vi "Prueba_report.vi"() -> ()   [LabVIEW 2025]
panel:
  out "Waveform Chart":dbl(graph)
  out "Waveform Graph":dbl[](graph)
  in  "stop":bool
  out "error out":errorcluster
  in  "error in (no error)":errorcluster
  in  "Canal 3":string
  in  "Canal 2":string
  in  "Canal 1":string
  in  "Grupo":string
  in  "Cantidad de datos":i32
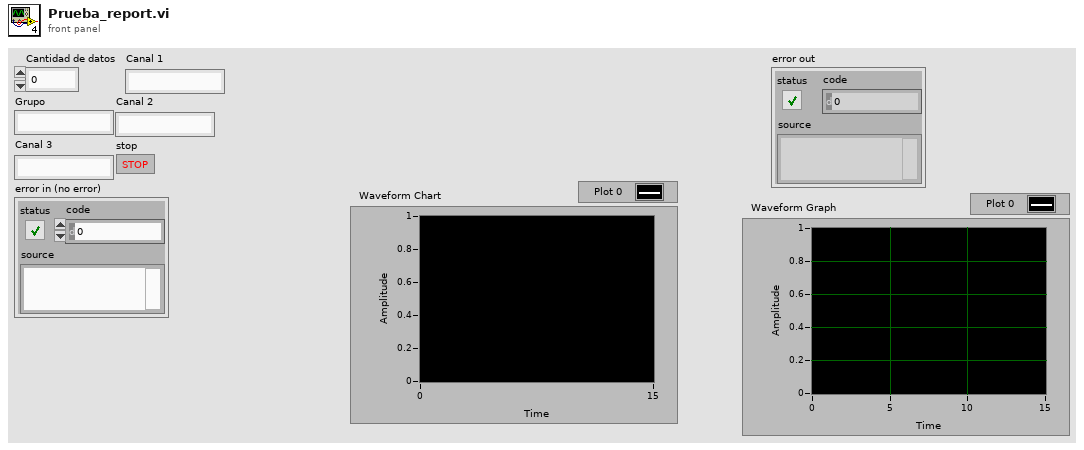
[diagram p1: front panel]
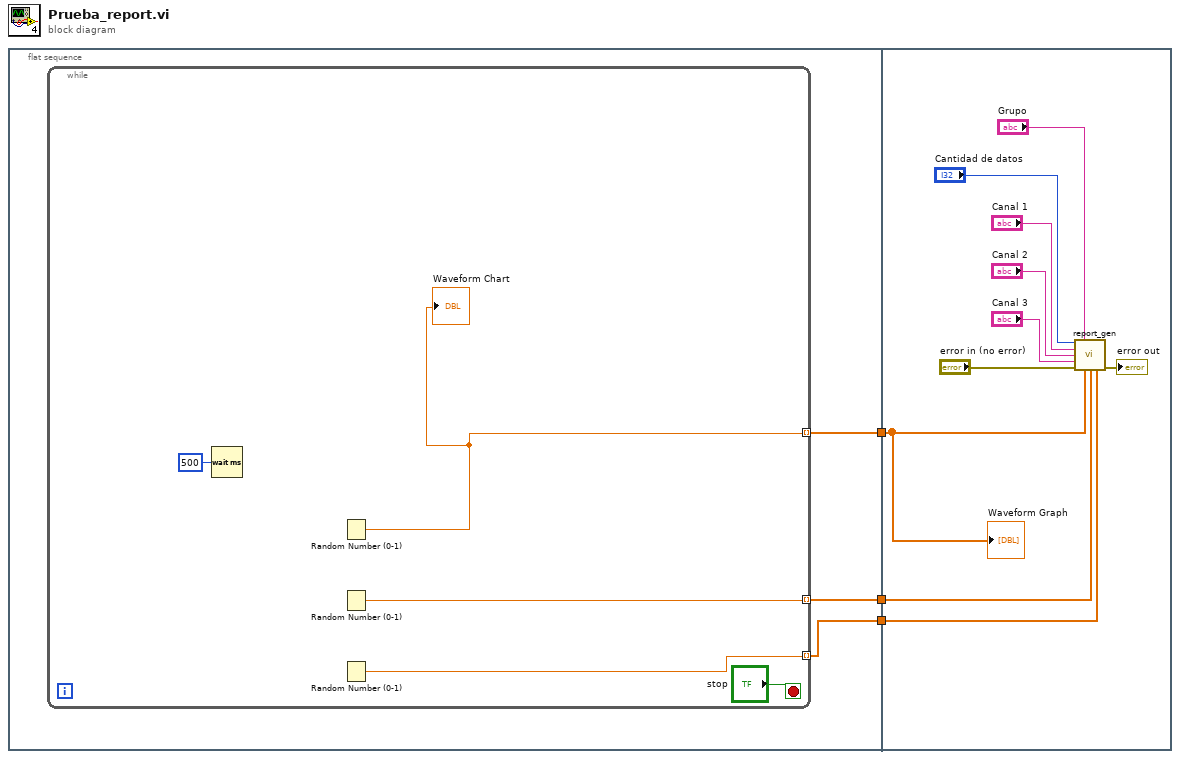
[diagram p0: block diagram]
diagram:
  n1 = flat-sequence {
    tunnel: [w6] -> w3
    tunnel: [w5] -> w2
    tunnel: [w4] -> w1
    tunnel: w3 -> [w13]
    tunnel: w2 -> [w12]
    tunnel: w1 -> [w14]
    frame #0 {
      n2 = while {
        tunnel: [w7] -> w4 mode=indexing
        tunnel: [w9] -> w6 mode=indexing
        tunnel: [w8] -> w5 mode=indexing
        stop <- "stop" stop-if-true
        n3 = Wait (ms)(milliseconds to wait=u32 500) -> ()  [unwired: 1 out]
        n4 = Random Number (0-1)() -> (number: 0 to 1=w7:dbl)
        "Waveform Chart" <- w7
        n5 = Random Number (0-1)() -> (number: 0 to 1=w9:dbl)
        n6 = Random Number (0-1)() -> (number: 0 to 1=w8:dbl)
      }
    }
    frame #1 {
      n7 = call "report_gen.vi"("Cantidad de datos"="Cantidad de datos", "Grupo"="Grupo", "Canal 1"="Canal 1", "Canal 2"="Canal 2", "Canal 3"="Canal 3", "error in (no error)"="error in (no error)", "Sensor 1"=w14, "Sensor 2"=w13, "Sensor 3"=w12) -> ("error out"=→"error out":errorcluster)  [unwired: 6 in]
      "Waveform Graph" <- w14
    }
  }
